vi "solar_log Variant to String.vi"(6 "ArrayDelimiters (1D,2D)":string[](array[string]), 8 "error in (no error)":errorcluster, 9 "Boolean as 0,1? (F)":bool, 10 "Use Enum Names? (F)":bool, 11 "Variant":variant) -> (0 "error out":errorcluster, 2 "Quotes Recommended?":bool, 3 "String":string)   [LabVIEW 2018]
doc: "This flattens the variant data to a human readable comma delimited string.\nEx: 'VALUE1, VALUE2, ...'"
uses:
  <vilib>/Utility/Data Type/NI_Data Type.lvlib
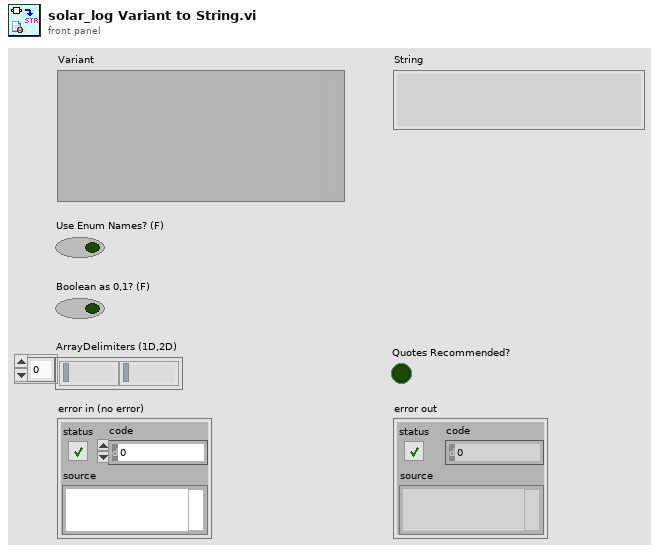
[diagram p1: front panel]
types:
  T1 = typedef "NI_Data Type.lvlib/Data Type.ctl" = enum8{"Invalid Type", "Void", "I8", "I16", "I32", "I64", "U8", "U16", "U32", "U64", "Single Float", "Double Float", "Extended Float", "Single Complex", "Double Complex", "Extended Complex", "Enum U8", "Enum U16", "Enum U32", "Enum U64", "Single Float With Unit", "Double Float With Unit", "Extended Float With Unit", "Single Complex with Unit", "Double Complex with Unit", "Extended Complex with Unit", "Boolean", "String", "Path", "Picture", "Tag", "Array", "Cluster", "Variant", "LV Variant", "Waveform", "Timestamp", "Digital Waveform", "Digital Data", "ExpressData", "Refnum", "External Data", "VI", "Poly VI", "LabVIEW Class Instance", "Fixed Point", "Set Collection", "Map Collection"}
  T2 = typedef "NI_Data Type.lvlib/Refnum Type.ctl" = enum16{"NotARefnum", "UnknownRefnum", "Generic", "Datalog", "ByteStream", "Device", "Occurence", "TCPNetConnection", "Auto", "Menu", "Imaq", "Hardware", "DataSocket", "Visa", "IVI", "UDPNetConnection", "Notifier", "Queue", "Irda", "EventReg", "DotNet", "UserEvent", "Callback", "UNUSED_EMPTY_POSITION", "BlueToothNetConnection", "LVObjApp", "LVObjVI", "LVObjUnknown", "GenericClass", "UserDefinedRefnumTag", "DataValue", "RT FIFO", "TDMS File", "PythonSessionRefnum"}
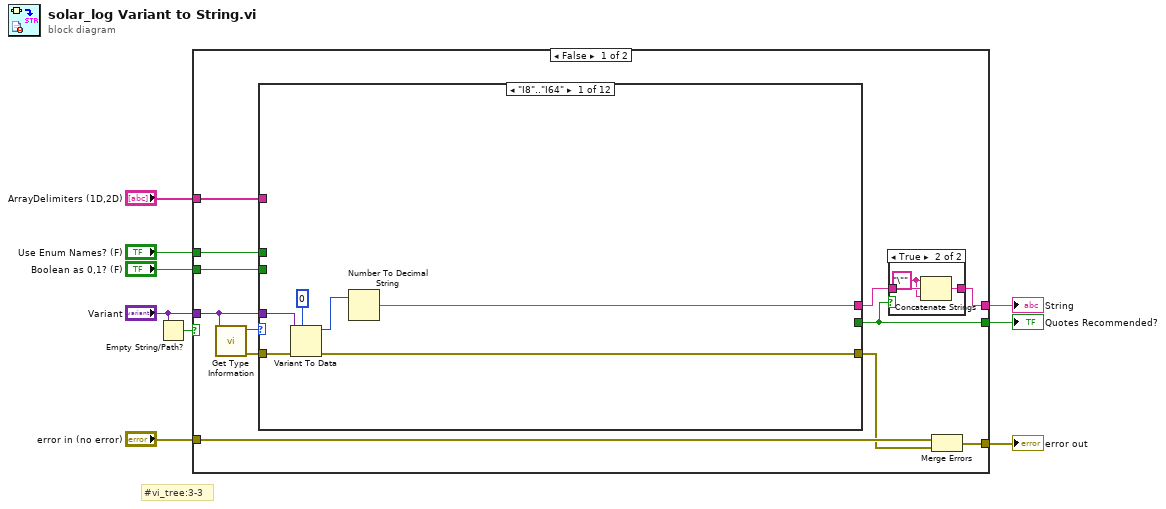
[diagram p0: block diagram]
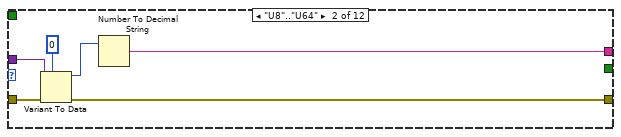
[diagram p3: hidden frame]
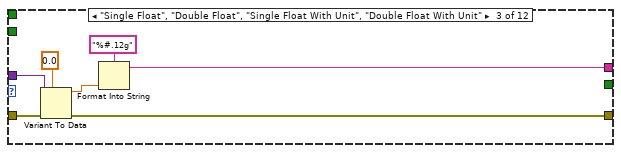
[diagram p4: hidden frame]
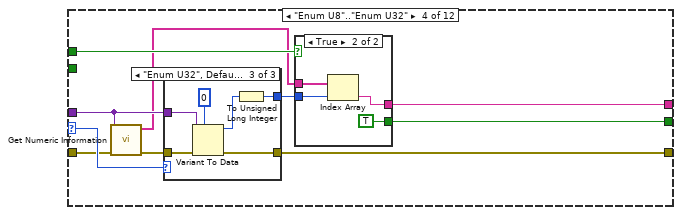
[diagram p5: hidden frame]
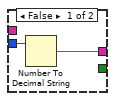
[diagram p6: hidden frame]
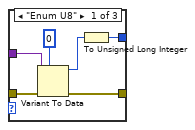
[diagram p7: hidden frame]
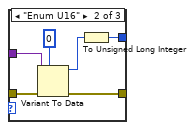
[diagram p8: hidden frame]
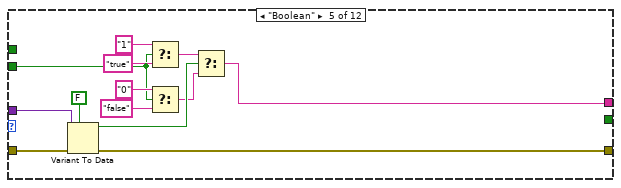
[diagram p9: hidden frame]
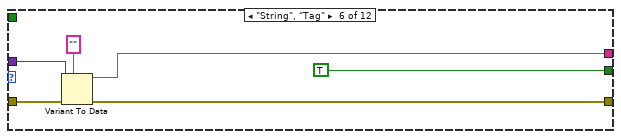
[diagram p10: hidden frame]
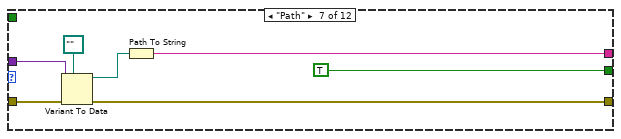
[diagram p11: hidden frame]
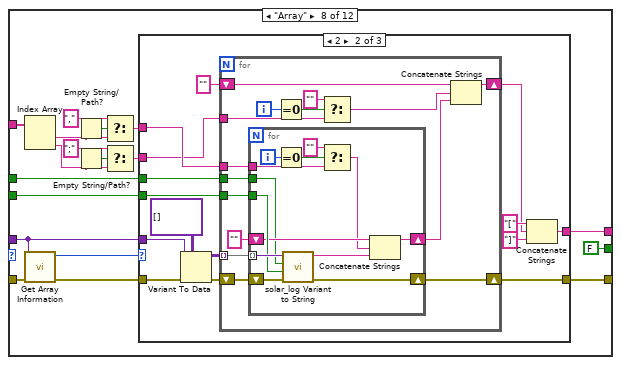
[diagram p12: hidden frame]
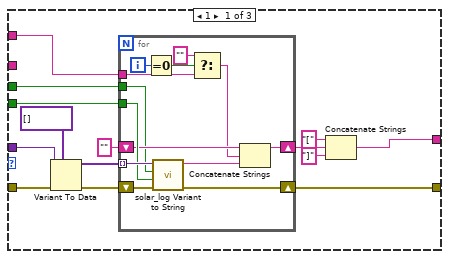
[diagram p13: hidden frame]
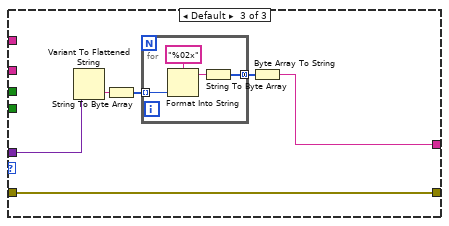
[diagram p14: hidden frame]
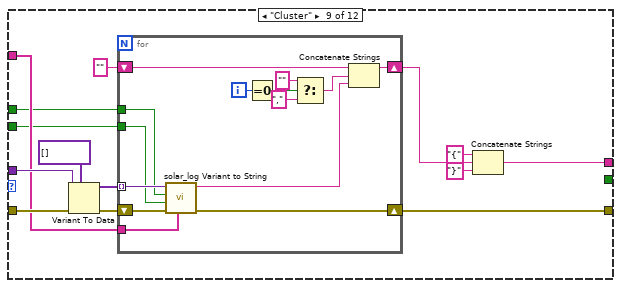
[diagram p15: hidden frame]
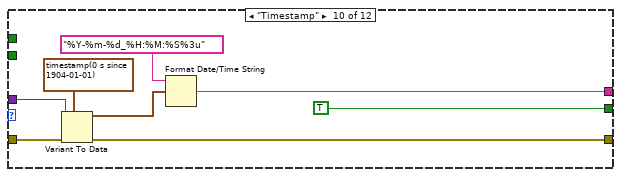
[diagram p16: hidden frame]
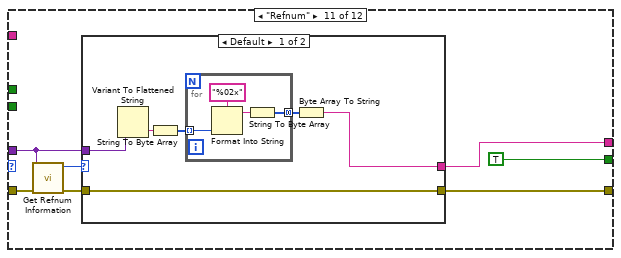
[diagram p17: hidden frame]
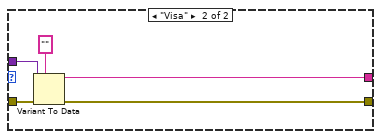
[diagram p18: hidden frame]
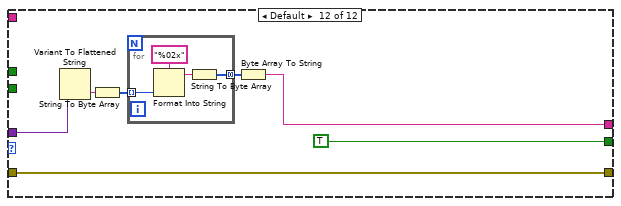
[diagram p19: hidden frame]
diagram:
  # "#vi_tree:3-3"
  n1 = Empty String/Path?(string/path="Variant") -> (empty?=w1:bool)
  n2 = case shown="False" w1 {
    tunnel: "Boolean as 0,1? (F)" -> [w19 _]
    tunnel: "Use Enum Names? (F)" -> [w18 _]
    tunnel: "ArrayDelimiters (1D,2D)" -> [w17 _]
    tunnel: "error in (no error)" -> [w16 w272]
    tunnel: [w14 w272] -> w5
    tunnel: [w10 _] -> w4
    tunnel: [w12 _] -> w3
    tunnel: "Variant" -> [w11 _]
    frame False {
      n3 = call <vilib>:"Get Type Information.vi"("variant"=w11) -> ("error out"=w20:errorcluster, "type"=w21:T1)  [unwired: 6 in, 3 out]
      n4 = case shown="\"I8\"..\"I64\"" w21 {
        selector: w21 -> [_ _ _ w51 _ _ _ _ _ _ _ _]
        tunnel: w11 -> [w30 w36 w43 w49 w82 w96 w103 w119 w215 w237 w242 w263]
        tunnel: w20 -> [w31 w37 w44 w50 w83 w97 w104 w122 w216 w238 w243 w267]
        tunnel: [w28 w34 w41 w54 w79 w94 w101 w108 w213 w236 w245 w267] -> w15
        tunnel: [w26 w32 w39 w52 w80 w93 w99 w107 w205 w233 w244 w262] -> w13
        tunnel: w19 -> [_ _ _ _ w81 _ _ w111 w208 _ _ _]
        tunnel: w18 -> [_ _ _ w47 _ _ _ w110 w209 _ _ _]
        tunnel: [_ _ _ w45 _ TRUE TRUE FALSE _ TRUE TRUE TRUE] -> w10
        tunnel: w17 -> [_ _ _ _ _ _ _ w116 w210 _ _ _]
        frame "I8".."I64" {
          n5 = Variant To Data(error in=w31, type=i64 0, Variant=w30) -> (data=w27:i64, error out=w28:errorcluster)
          n6 = Number To Decimal String(number=w27) -> (decimal integer string=w26:string)  [unwired: 1 in]
        }
        frame "U8".."U64" {
          n7 = Variant To Data(error in=w37, type=u64 0, Variant=w36) -> (data=w33:u64, error out=w34:errorcluster)
          n8 = Number To Decimal String(number=w33) -> (decimal integer string=w32:string)  [unwired: 1 in]
        }
        frame "Single Float", "Double Float", "Single Float With Unit", "Double Float With Unit" {
          n9 = Variant To Data(error in=w44, type=0.0, Variant=w43) -> (data=w40:dbl, error out=w41:errorcluster)
          n10 = Format Into String(format string="%#.12g", w40) -> (resulting string=w39:string)  [unwired: 2 in, 1 out]
        }
        frame "Enum U8".."Enum U32" {
          n11 = call <vilib>:"Get Numeric Information.vi"("error in (no error)"=w50, "variant"=w49) -> ("error out"=w48:errorcluster, "enum names"=w46:string[])  [unwired: 6 in, 2 out]
          n12 = case shown="\"Enum U32\", Default" w51 {
            tunnel: w48 -> [w66 w72 w78]
            tunnel: w49 -> [w65 w71 w77]
            tunnel: [w63 w69 w75] -> w54
            tunnel: [w61 w67 w73] -> w53
            frame "Enum U8" {
              n13 = Variant To Data(error in=w66, type=u8 0, Variant=w65) -> (data=w62:u8, error out=w63:errorcluster)
              n14 = To Unsigned Long Integer(number=w62) -> (unsigned 32bit integer=w61:u32)
            }
            frame "Enum U16" {
              n15 = Variant To Data(error in=w72, type=u16 0, Variant=w71) -> (data=w68:u16, error out=w69:errorcluster)
              n16 = To Unsigned Long Integer(number=w68) -> (unsigned 32bit integer=w67:u32)
            }
            frame "Enum U32", Default {
              n17 = Variant To Data(error in=w78, type=u32 0, Variant=w77) -> (data=w74:u32, error out=w75:errorcluster)
              n18 = To Unsigned Long Integer(number=w74) -> (unsigned 32bit integer=w73:u32)
            }
          }
          n19 = case shown="True" w47 {
            tunnel: w53 -> [w56 w60]
            tunnel: [w55 w58] -> w52
            tunnel: w46 -> [_ w59]
            tunnel: [_ TRUE] -> w45
            frame False {
              n20 = Number To Decimal String(number=w56) -> (decimal integer string=w55:string)  [unwired: 1 in]
            }
            frame True {
              n21 = Index Array(array=w59, index=w60) -> (element=w58:string)
            }
          }
        }
        frame "Boolean" {
          n22 = Variant To Data(error in=w83, type=FALSE, Variant=w82) -> (data=w90:bool, error out=w79:errorcluster)
          n23 = Select(t="1", s=w81, f="true") -> (s? t:f=w85:string)
          n24 = Select(t="0", s=w81, f="false") -> (s? t:f=w84:string)
          n25 = Select(t=w85, s=w90, f=w84) -> (s? t:f=w80:string)
        }
        frame "String", "Tag" {
          n26 = Variant To Data(error in=w97, type="", Variant=w96) -> (data=w93:string, error out=w94:errorcluster)
        }
        frame "Path" {
          n27 = Variant To Data(error in=w104, type=path "", Variant=w103) -> (data=w100:path, error out=w101:errorcluster)
          n28 = Path To String(path=w100) -> (string=w99:string)
        }
        frame "Array" {
          n29 = Index Array(array=w116) -> (element #1=w117:string, element #2=w115:string)  [unwired: 2 in]
          n30 = call <vilib>:"Get Array Information.vi"("error in (no error)"=w122, "variant"=w119) -> ("error out"=w120:errorcluster, "number of dimensions"=w121:i32)  [unwired: 6 in, 2 out]
          n31 = Empty String/Path?(string/path=w117) -> (empty?=w118:bool)
          n32 = Empty String/Path?(string/path=w115) -> (empty?=w113:bool)
          n33 = Select(t=",", s=w118, f=w117) -> (s? t:f=w109:string)
          n34 = Select(t=";", s=w113, f=w115) -> (s? t:f=w105:string)
          n35 = case shown="2" w121 {
            tunnel: w120 -> [w136 w164 w193]
            tunnel: w119 -> [w135 w163 w195]
            tunnel: w111 -> [w131 w159 _]
            tunnel: w110 -> [w130 w158 _]
            tunnel: w109 -> [w129 w157 _]
            tunnel: [w128 w156 w193] -> w108
            tunnel: [w125 w150 w194] -> w107
            tunnel: w105 -> [_ w155 _]
            frame 1 {
              n36 = Variant To Data(error in=w136, type=variant[] [], Variant=w135) -> (data=w132:variant[], error out=w133:errorcluster)
              n37 = for {
                tunnel: w132 -> [w148] mode=indexing
                tunnel: w131 -> [w147]
                tunnel: w130 -> [w137]
                shift-right: [w145] -> w126
                shift-left: "" -> [w144]
                tunnel: w129 -> [w140]
                shift-right: [w143] -> w128
                shift-left: w133 -> [w149]
                i -> [w142]
                n38 = Equal To 0?(x=w142) -> (x = 0?=w141:bool)
                n39 = call "solar_log Variant to String.vi"("error in (no error)"=w149, "Boolean as 0,1? (F)"=w147, "Use Enum Names? (F)"=w137, "Variant"=w148) -> ("error out"=w143:errorcluster, "String"=w146:string)  [unwired: 5 in, 1 out]
                n40 = Select(t="", s=w141, f=w140) -> (s? t:f=w139:string)
                n41 = Concatenate Strings(w144, w139, w146) -> (w145:string)
              }
              n42 = Concatenate Strings("[" ("string"), w126, "]" ("string")) -> (w125:string)
            }
            frame 2 {
              n43 = Variant To Data(error in=w164, type=variant[][] [], Variant=w163) -> (data=w160:variant[][], error out=w161:errorcluster)
              n44 = for {
                tunnel: w160 -> [w178] mode=indexing
                tunnel: w159 -> [w177]
                tunnel: w158 -> [w176]
                tunnel: w157 -> [w174]
                shift-right: [w173] -> w156
                shift-left: w161 -> [w179]
                tunnel: w155 -> [w169]
                shift-right: [w166] -> w151
                shift-left: "" -> [w165]
                i -> [w170]
                n45 = for {
                  tunnel: w178 -> [w191] mode=indexing
                  tunnel: w177 -> [w190]
                  tunnel: w176 -> [w180]
                  shift-right: [w188] -> w172
                  shift-left: "" -> [w187]
                  tunnel: w174 -> [w183]
                  shift-right: [w186] -> w173
                  shift-left: w179 -> [w192]
                  i -> [w185]
                  n46 = Equal To 0?(x=w185) -> (x = 0?=w184:bool)
                  n47 = call "solar_log Variant to String.vi"("error in (no error)"=w192, "Boolean as 0,1? (F)"=w190, "Use Enum Names? (F)"=w180, "Variant"=w191) -> ("error out"=w186:errorcluster, "String"=w189:string)  [unwired: 5 in, 1 out]
                  n48 = Select(t="", s=w184, f=w183) -> (s? t:f=w182:string)
                  n49 = Concatenate Strings(w187, w182, w189) -> (w188:string)
                }
                n50 = Equal To 0?(x=w170) -> (x = 0?=w171:bool)
                n51 = Select(t="", s=w171, f=w169) -> (s? t:f=w167:string)
                n52 = Concatenate Strings(w165, w167, w172) -> (w166:string)
              }
              n53 = Concatenate Strings("[" ("string"), w151, "]" ("string")) -> (w150:string)
            }
            frame Default {
              n54 = Variant To Flattened String(Variant=w195) -> (data string=w196:string)  [unwired: 1 out]
              n55 = String To Byte Array(string=w196) -> (unsigned byte array=w198:u8[])
              n56 = for {
                tunnel: w198 -> [w202] mode=indexing
                tunnel: [w199] -> w197 mode=concatenating
                n57 = Format Into String(format string="%02x" ("Format String"), w202) -> (resulting string=w200:string)  [unwired: 2 in, 1 out]
                n58 = String To Byte Array(string=w200) -> (unsigned byte array=w199:u8[])
              }
              n59 = Byte Array To String(unsigned byte array=w197) -> (string=w194:string)
            }
          }
        }
        frame "Cluster" {
          n60 = Variant To Data(error in=w216, type=variant[] [], Variant=w215) -> (data=w211:variant[], error out=w212:errorcluster)
          n61 = for {
            shift-right: [w229] -> w213
            shift-left: w212 -> [w230]
            tunnel: w211 -> [w227] mode=indexing
            tunnel: w210 -> [w228]
            tunnel: w209 -> [w226]
            tunnel: w208 -> [w225]
            shift-right: [w218] -> w206
            shift-left: "" -> [w224]
            i -> [w223]
            n62 = call "solar_log Variant to String.vi"("ArrayDelimiters (1D,2D)"=w228, "error in (no error)"=w230, "Boolean as 0,1? (F)"=w225, "Use Enum Names? (F)"=w226, "Variant"=w227) -> ("error out"=w229:errorcluster, "String"=w217:string)  [unwired: 4 in, 1 out]
            n63 = Equal To 0?(x=w223) -> (x = 0?=w222:bool)
            n64 = Select(t="", s=w222, f=",") -> (s? t:f=w219:string)
            n65 = Concatenate Strings(w224, w219, w217) -> (w218:string)
          }
          n66 = Concatenate Strings("{" ("string"), w206, "}" ("string")) -> (w205:string)
        }
        frame "Timestamp" {
          n67 = Variant To Data(error in=w238, type=timestamp(0 s since 1904-01-01), Variant=w237) -> (data=w234:timestamp, error out=w236:errorcluster)
          n68 = Format Date/Time String(time format string (%c)="%Y-%m-%d_%H:%M:%S%3u", seconds (now)=w234) -> (date/time string=w233:string)  [unwired: 1 in]
        }
        frame "Refnum" {
          n69 = call <vilib>:"Get Refnum Information.vi"("error in (no error)"=w243, "variant"=w242) -> ("error out"=w241:errorcluster, "reference type"=w240:T2)  [unwired: 6 in, 2 out]
          n70 = case shown="Default" w240 {
            tunnel: [w251 w259] -> w245
            tunnel: [w246 w258] -> w244
            tunnel: w242 -> [w247 w257]
            tunnel: w241 -> [w251 w256]
            frame Default {
              n71 = Variant To Flattened String(Variant=w247) -> (data string=w248:string)  [unwired: 1 out]
              n72 = String To Byte Array(string=w248) -> (unsigned byte array=w250:u8[])
              n73 = for {
                tunnel: w250 -> [w255] mode=indexing
                tunnel: [w252] -> w249 mode=concatenating
                n74 = Format Into String(format string="%02x" ("Format String"), w255) -> (resulting string=w253:string)  [unwired: 2 in, 1 out]
                n75 = String To Byte Array(string=w253) -> (unsigned byte array=w252:u8[])
              }
              n76 = Byte Array To String(unsigned byte array=w249) -> (string=w246:string)
            }
            frame "Visa" {
              n77 = Variant To Data(error in=w256, type="", Variant=w257) -> (data=w258:string, error out=w259:errorcluster)
            }
          }
        }
        frame Default {
          n78 = Variant To Flattened String(Variant=w263) -> (data string=w264:string)  [unwired: 1 out]
          n79 = String To Byte Array(string=w264) -> (unsigned byte array=w266:u8[])
          n80 = for {
            tunnel: w266 -> [w271] mode=indexing
            tunnel: [w268] -> w265 mode=concatenating
            n81 = Format Into String(format string="%02x" ("Format String"), w271) -> (resulting string=w269:string)  [unwired: 2 in, 1 out]
            n82 = String To Byte Array(string=w269) -> (unsigned byte array=w268:u8[])
          }
          n83 = Byte Array To String(unsigned byte array=w265) -> (string=w262:string)
        }
      }
      n84 = case shown="True" w10 {
        tunnel: w13 -> [w22 w25]
        tunnel: [w22 w23] -> w12
        frame False {
        }
        frame True {
          w24 = "\"" ("string")
          n85 = Concatenate Strings(w24, w25, w24) -> (w23:string)
        }
      }
      n86 = Merge Errors(w16, w15) -> (w14:errorcluster)
    }
    frame True {
    }
  }
  "String" <- w3
  "error out" <- w5
  "Quotes Recommended?" <- w4
